vi "Initialize.vi"(8 "error in":errorcluster, 11 "session in":refnum<class "Session.lvclass">) -> (0 "error out":errorcluster, 3 "session out":refnum<class "Session.lvclass">)   [LabVIEW 2020, in "NI_SFTP.lvlib" / "Session.lvclass"]
uses:
  <vilib>/net/SFTP/Session/Session.lvclass
  <vilib>/net/SFTP/Session/Handle.ctl
  <vilib>/net/SFTP/Session/Session.lvclass/Session.ctl
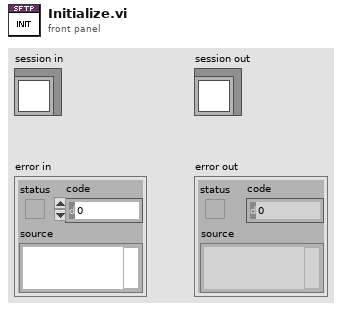
[diagram p1: front panel]
types:
  T1 = typedef "NI_SFTP.lvlib/Session.lvclass/Handle.ctl" = u8[]
  T2 = typedef "Semaphore RefNum" = refnum<k1>
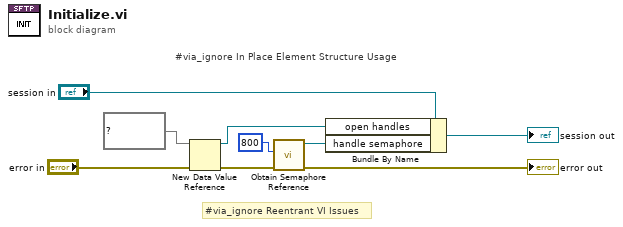
[diagram p0: block diagram]
diagram:
  # "#via_ignore Reentrant VI Issues"
  # "#via_ignore In Place Element Structure Usage"
  n1 = New Data Value Reference(data value=set{T1} {} ("ids"), error in="error in") -> (data value reference=w6:refnum<data-value>, error out=w5:errorcluster)
  n2 = call <vilib>:"Obtain Semaphore Reference.vi"("error in (no error)"=w5, "size (1)"=800) -> ("error out"=→"error out":errorcluster, "semaphore"=w3:T2)  [unwired: 3 in, 1 out]
  n3 = Bundle By Name(cluster="session in", "open handles"=w6, "handle semaphore"=w3) -> (→"session out":refnum<class "Session.lvclass">)
